vi "S2C_FORNAX_Proc_FindValue.vi"(8 "Error In":errorcluster, 9 "Row":i32, 10 "CtlRef":refnum<vi>, 11 "ItemTag":string) -> (0 "Error Out":errorcluster, 2 "Found?":bool, 3 "Value_Int":string)   [LabVIEW 2015]
doc: "Finds the Int value for a selected Fornax command type."
uses:
  S2C_FORNAX_Proc_Globals.vi
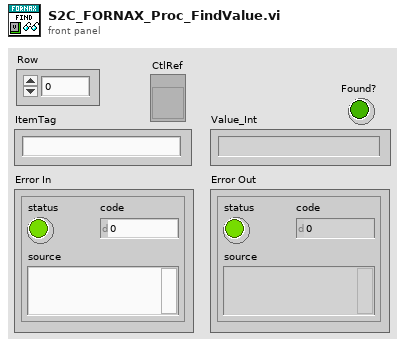
[diagram p1: front panel]
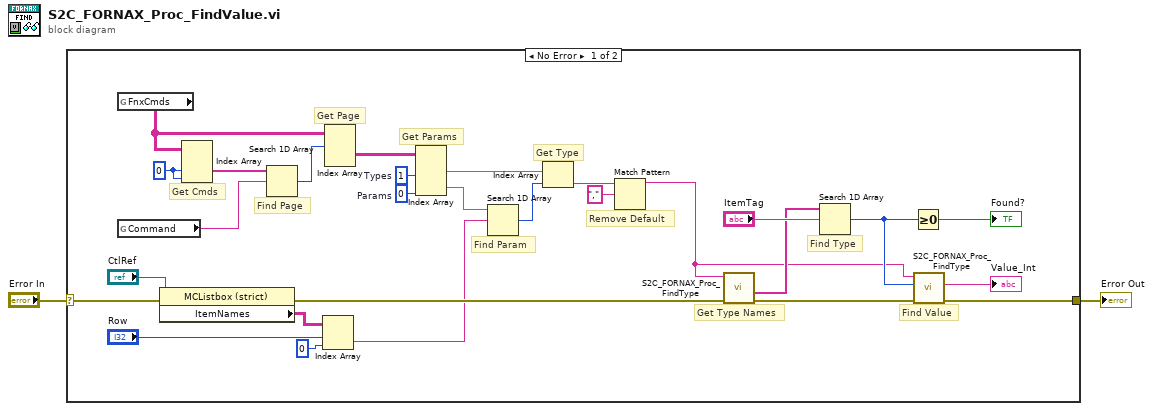
[diagram p0: block diagram]
diagram:
  n1 = case shown="No Error" "Error In" {
    selector: "Error In" -> [w30 w31]
    tunnel: [w24 w31] -> w1
    frame No Error {
      w17 = 0  # Params
      w18 = 1  # Types
      w21 = 0 ("disabled index (row)")
      # "Remove Default"
      # "Find Value"
      # "Find Type"
      # "Get Type Names"
      # "Get Type"
      # "Find Param"
      # "Get Params"
      # "Get Page"
      # "Find Page"
      # "Get Cmds"
      n2 = global read "S2C_FORNAX_Proc_Globals.vi" "FnxCmds"() -> (w4:string[][][])
      n3 = global read "S2C_FORNAX_Proc_Globals.vi" "Command"() -> (w3:string)
      n4 = property class="MCListbox (strict)"(reference="CtlRef", error in=w30) -> (error out=w25:errorcluster, "ItemNames"=w28:string[][])  [unwired: 1 out]
      n5 = Index Array(array=w4, index (dim 1)=w21, index (dim 2)=w21) -> (element=w22:string[])  [unwired: 1 in]
      n6 = Search 1D Array(1D array=w22, element=w3) -> (index of element=w20:i32)  [unwired: 1 in]
      n7 = Index Array(array=w28, index (row)="Row", index (col)=0 ("disabled index (col)")) -> (element=w8:string)
      n8 = Index Array(array=w4, index (dim 0)=w20) -> (element=w19:string[][])  [unwired: 2 in]
      n9 = Index Array(array=w19, index (col) #1=w18, index (col) #2=w17) -> (element #1=w15:string[], element #2=w16:string[])  [unwired: 2 in]
      n10 = Search 1D Array(1D array=w16, element=w8) -> (index of element=w14:i32)  [unwired: 1 in]
      n11 = Index Array(array=w15, index=w14) -> (element=w7:string)
      n12 = Match Pattern(string=w7, regular expression=",") -> (before substring=w5:string)  [unwired: 1 in, 3 out]
      n13 = call "S2C_FORNAX_Proc_FindType.vi"("Error In"=w25, "TypeString"=w5) -> ("Error Out"=w10:errorcluster, "AllValues"=w11:string[])  [unwired: 5 in, 3 out]
      n14 = Search 1D Array(1D array=w11, element="ItemTag") -> (index of element=w9:i32)  [unwired: 1 in]
      n15 = Greater Or Equal To 0?(x=w9) -> (x >= 0?=→"Found?":bool)
      n16 = call "S2C_FORNAX_Proc_FindType.vi"("Error In"=w10, "Index"=w9, "TypeString"=w5) -> ("Error Out"=w24:errorcluster, "Value_Int"=→"Value_Int":string)  [unwired: 4 in, 3 out]
    }
    frame Error {
    }
  }
  "Error Out" <- w1
